vi "Start.vi"(8 "error in":errorcluster, 11 "Tx Acyclic Execution Unit in":refnum<class "Tx Acyclic Labels Execution Unit.lvclass">) -> (0 "error out":errorcluster, 3 "Tx Acyclic Execution Unit out":refnum<class "Tx Acyclic Labels Execution Unit.lvclass">)   [LabVIEW 2020, in "AIM ARINC 429 Engine.lvlib" / "Implementation.lvlib" / "Tx Acyclic Labels Execution Unit.lvclass"]
uses:
  Tx Acyclic Labels Execution Unit.lvclass
  Hardware API/AIM ARINC 429 Hardware API.lvlib
  Execution Unit/Execution Unit.lvclass
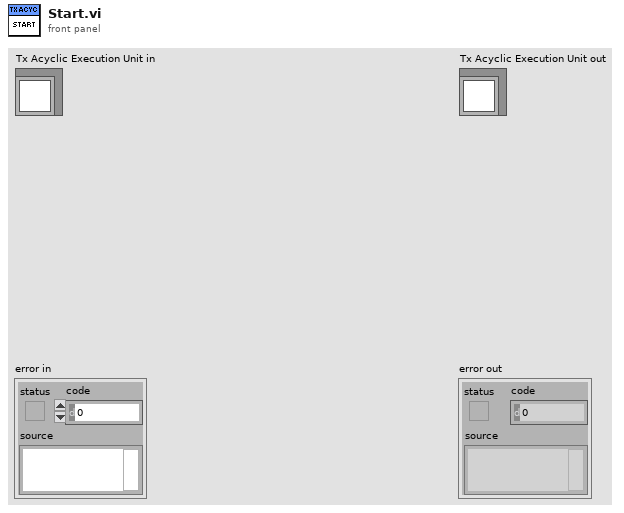
[diagram p1: front panel]
types:
  T1 = typedef "RT Hardware Channel Settings.ctl" = cluster{"channel #":u16, "channel handle":u64, "labels settings for RT":T2[]}
  T2 = typedef "RT Label Settings.ctl" = cluster{"Name":string, "xmlName":string, "label":T3, "transfer period":u32, "SDI_Enabled":bool, "SDI":u8, "parameter driver data":T4, "transfer type":T8, "has timestamp?":bool, "Label Disable/Trigger Channel Reference":T7, "Message Handle":u64, "Initialized?":bool, "Word Initial Raw Value":u32, "Label Timestamp Channel Data Reference":T9, "disabled":bool}
  T3 = typedef "Label.ctl" = u8
  T4 = typedef "RT Parameters.ctl" = cluster{"parameter definitions":T5[], "Tx parameter refs":T7[]}
  T5 = typedef "Parameter Definition.ctl" = cluster{"start index":i32, "size":i32, "encoding":T6, "signed":bool, "scale multiplier":dbl, "scale offset":dbl, "default value":dbl}
  T6 = typedef "Encoding and Decoding.lvlib/Encoding.ctl" = enum16{"BNR", "BCD", "Discrete"}
  T7 = typedef "Custom Device API.lvlib/Custom Device Item Ref.ctl" = u64
  T8 = typedef "Transfer Type.ctl" = enum16{"Scheduled", "Acyclic", "Block", "Strobe"}
  T9 = typedef "Custom Device API.lvlib/Data Reference.ctl" = i32
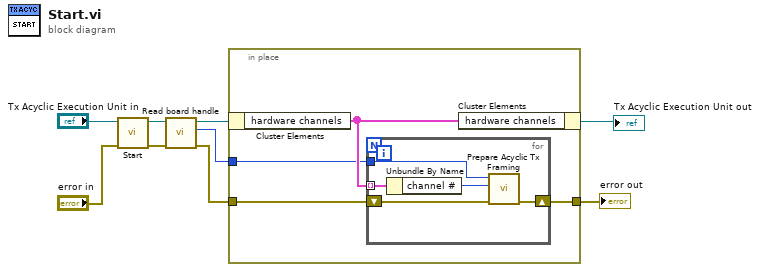
[diagram p0: block diagram]
diagram:
  n1 = call-parent "Start.vi"("error in"="error in", "Execution Unit Implementation in"="Tx Acyclic Execution Unit in") -> ("error out"=w5:errorcluster, "Execution Unit Implementation out"=w3:refnum<class "Tx Acyclic Labels Execution Unit.lvclass">)  [unwired: 8 in]
  n2 = call "Read board handle.vi"("error in (no error)"=w5, "Execution Unit in"=w3) -> ("error out"=w4:errorcluster, "board handle"=w1:u8, "Execution Unit out"=w2:refnum<class "Tx Acyclic Labels Execution Unit.lvclass">)  [unwired: 7 in]
  n3 = in-place {
    in-place-border: w4 -> [w11]
    in-place-border: [w10] -> w6
    in-place-border: w1 -> [w12]
    n4 = in-place-cluster #1(w2) -> ("hardware channels"=w13:T1[])
    n5 = for {
      tunnel: w13 -> [w18] mode=indexing
      tunnel: w12 -> [w16]
      shift-right: [w14] -> w10
      shift-left: w11 -> [w15]
      n6 = Unbundle By Name(w18) -> ("channel #"=w17:u16)
      n7 = call "Prepare Acyclic Tx Framing.vi"("error in"=w15, "channel number in"=w17, "board handle in"=w16) -> ("error out"=w14:errorcluster)  [unwired: 6 in, 2 out]
    }
    n8 = in-place-cluster #1("hardware channels"=w13) -> (→"Tx Acyclic Execution Unit out":refnum<class "Tx Acyclic Labels Execution Unit.lvclass">)
  }
  "error out" <- w6
